vi "Read Global Locked.vi"(7 "Semaphore Timeout":i32=-1, 8 "error in (no error)":errorcluster, 11 "System in":refnum<class "System.lvclass">) -> (0 "error out":errorcluster, 1 "Semaphore Timed Out":bool, 2 "Global":refnum<class "System.lvclass">, 3 "System out":refnum<class "System.lvclass">)   [LabVIEW 2013, in "System.lvclass"]
uses:
  System.lvclass
  System.lvclass/System.ctl
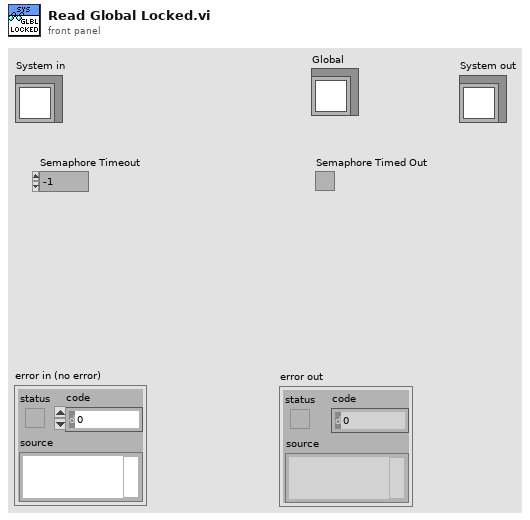
[diagram p1: front panel]
types:
  T1 = typedef "Semaphore RefNum" = refnum<k1>
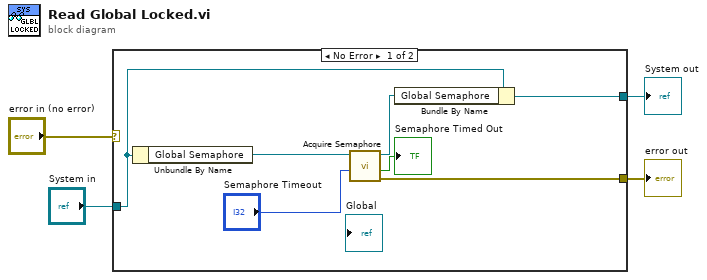
[diagram p0: block diagram]
diagram:
  n1 = case shown="No Error" "error in (no error)" {
    selector: "error in (no error)" -> [_ w13]
    tunnel: [w7 w13] -> w3
    tunnel: [w9 w12] -> w1
    tunnel: "System in" -> [w6 w12]
    frame No Error {
      n2 = Unbundle By Name(w6) -> ("Global Semaphore"=w5:T1)
      n3 = call <vilib>:"Acquire Semaphore.vi"("ms timeout (-1)"="Semaphore Timeout", "semaphore"=w5) -> ("error out"=w7:errorcluster, "timed out"=→"Semaphore Timed Out":bool, "semaphore out"=w8:T1)  [unwired: 3 in]
      n4 = Bundle By Name(cluster=w6, "Global Semaphore"=w8) -> (w9:refnum<class "System.lvclass">)
    }
    frame Error {
    }
  }
  "error out" <- w3
  "System out" <- w1
